vi "FITS - Format FITS Keyword.vi"(0 "Keyword":string="BITPIX", 1 "Value":string="16", 2 "Comment":string="BITS PER PIXEL") -> (3 "Formatted fits entry":string="BITPIX  =                   16 / BITS PER PIXEL                                 ", 5 "Length of line":i16=80)   [LabVIEW 2014]
uses:
  <vilib>/regexp/Match Regular Expression.xnode
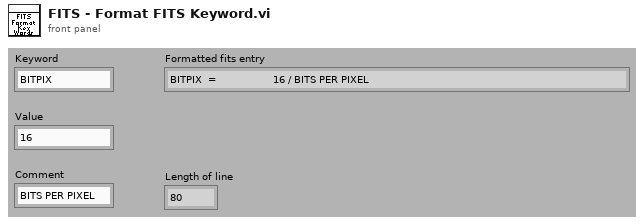
[diagram p1: front panel]
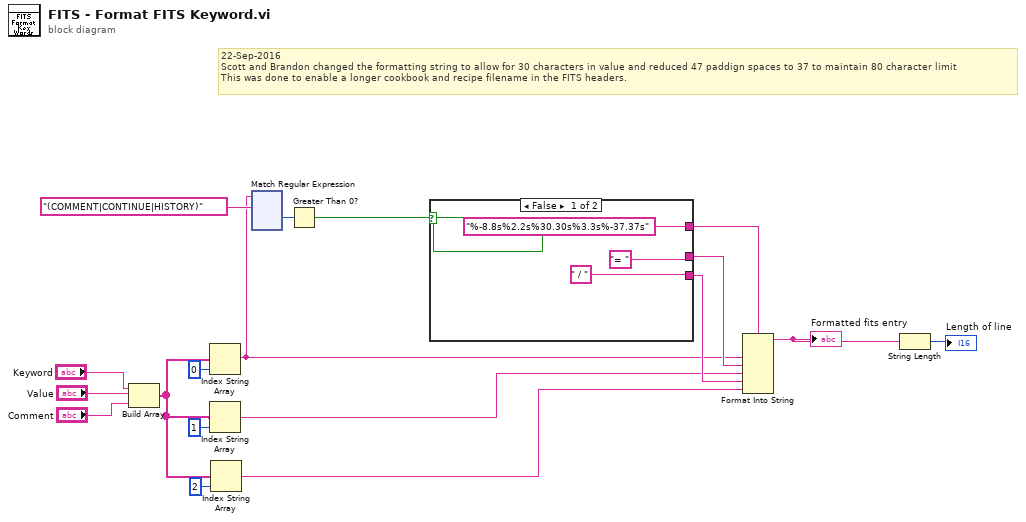
[diagram p0: block diagram]
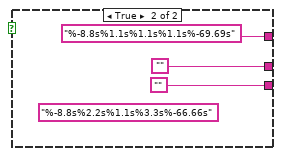
[diagram p2: hidden frame]
diagram:
  # "22-Sep-2016\nScott and Brandon changed the formatting string to allow for 30 characters in value and reduced 47 paddign spaces to 37 to maintain 80 character limit\nThis was done to enable a longer cookbook and recipe filename in the FITS headers."
  n1 = Build Array("Keyword", "Value", "Comment") -> (w15:string[])
  n2 = Index String Array(1:0 ("index"), 2:w15) -> (0:w2:string)  [unwired: 1 out]
  n3 = Index String Array(1:1 ("index"), 2:w15) -> (0:w7:string)  [unwired: 1 out]
  n4 = Index String Array(1:2 ("index"), 2:w15) -> (0:w9:string)  [unwired: 1 out]
  n5 = xnode "Match Regular Expression"("input string"=w2, "regular expression"="(COMMENT|CONTINUE|HISTORY)" ("true string")) -> ("offset past match"=w1:i32)  [unwired: 4 in, 4 out]
  n6 = Greater Than 0?(x=w1) -> (x > 0?=w13:bool)
  n7 = case shown="False" w13 {
    tunnel: ["= " ""] -> w12
    tunnel: [" / " ""] -> w11
    tunnel: ["%-8.8s%2.2s%30.30s%3.3s%-37.37s" ("format string") "%-8.8s%1.1s%1.1s%1.1s%-69.69s" ("format string")] -> w14
    frame False {
    }
    frame True {
      (unwired) "%-8.8s%2.2s%1.1s%3.3s%-66.66s" ("format string")
    }
  }
  n8 = Format Into String(format string=w14, w2, w12, w7, w11, w9) -> (resulting string=w3:string)  [unwired: 2 in, 1 out]
  "Formatted fits entry" <- w3
  n9 = String Length(string=w3) -> (length=→"Length of line":i32)
